vi "libssh2_session_callback_set.vi"(8 "error in (no error)":errorcluster, 9 "callback (0 = use built-in)":u64, 10 "callback type":T1, 11 "session":T2) -> (0 "error out":errorcluster, 2 "previous callback":u64)   [LabVIEW 2017, in "libssh2.lvlib"]
doc: "<B>DEPRECATED</B> (libssh2-1.11.1, use libssh2_session_callback_set2.vi)\n\nSet a callback handler for a session. Callbacks are triggered by the receipt of special packets at the transport layer.\n\nSet <B>callback</B> to 0 to to use the built-in default callback handler of lvssh2 (only available when the extension library is enabled). When the extension library is disabled, setting <B>callback</B> to 0 will disable the callback handler."
uses:
  libssh2.lvlib
  Session Refnum.ctl
  libssh2_session_callback_type.ctl
  Not A Session.vi
  <vilib>/Utility/error.llb/Error Cluster From Error Code.vi
  Global Settings.vi
  Read Session Refnum.vi
  <vilib>/Utility/semaphor.llb/Acquire Semaphore.vi
  <vilib>/Utility/semaphor.llb/Release Semaphore.vi
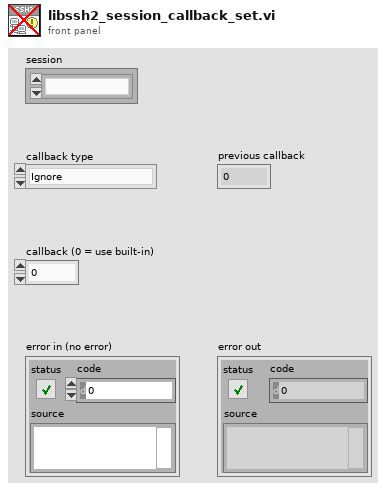
[diagram p1: front panel]
types:
  T1 = typedef "libssh2.lvlib/libssh2_session_callback_type.ctl" = enum16{"Ignore", "Debug", "Disconnect", "MAC Error", "X11", "Send", "Receive", "Auth Agent", "Auth Agent Identities", "Auth Agent Sign"}
  T2 = typedef "libssh2.lvlib/Session Refnum.ctl" = refnum<k1>
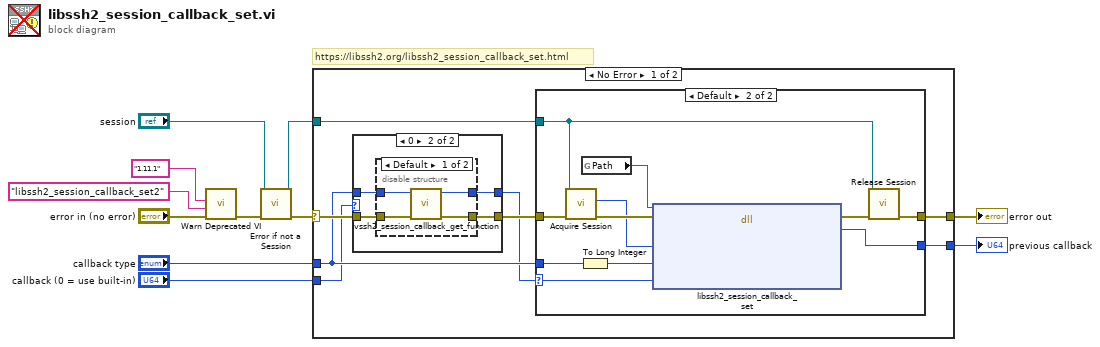
[diagram p0: block diagram]
diagram:
  # "https://libssh2.org/libssh2_session_callback_set.html"
  n1 = call "Warn Deprecated VI.vi"("error in (no error)"="error in (no error)", "replacement"="libssh2_session_callback_set2", "deprecated version"="1.11.1") -> ("error out"=w1:errorcluster)  [unwired: 8 in]
  n2 = call "Error if not a Session.vi"("error in (no error)"=w1, "session"="session") -> ("error out"=w6:errorcluster, "session out"=w5:T2)  [unwired: 8 in]
  n3 = case shown="No Error" w6 {
    selector: w6 -> [w19 w44]
    tunnel: [w13 w44] -> w11
    tunnel: w5 -> [w12 _]
    tunnel: "callback type" -> [w17 _]
    tunnel: [w16 _] -> w8
    tunnel: "callback (0 = use built-in)" -> [w14 _]
    frame No Error {
      n4 = case shown="0" w14 {
        selector: w14 -> [w33 _]
        tunnel: w19 -> [w32 w37]
        tunnel: [w32 w36] -> w18
        tunnel: w17 -> [_ w35]
        tunnel: [w33 w34] -> w15
        frame Default {
        }
        frame 0 {
          n5 = disable-structure shown="Default" {
            disable-tunnel: w37 -> [w41 w42]
            disable-tunnel: [w40 w42] -> w36
            disable-tunnel: w35 -> [w39 w43]
            disable-tunnel: [w38 w43] -> w34
            frame condition #0 (active) {
              n6 = call "lvssh2_session_callback_get_function.vi"("error in (no error)"=w41, "callback type"=w39) -> ("error out"=w40:errorcluster, "callback function"=w38:u64)  [unwired: 8 in]
            }
            frame condition #1 {
            }
          }
        }
      }
      n7 = case shown="Default" w15 {
        selector: w15 -> [_ w23]
        tunnel: w18 -> [w20 w27]
        tunnel: w17 -> [_ w26]
        tunnel: [_ w24] -> w16
        tunnel: [w20 w22] -> w13
        tunnel: w12 -> [_ w21]
        frame 0 {
        }
        frame Default {
          n8 = call "Acquire Session.vi"("error in (no error)"=w27, "session"=w21) -> ("error out"=w31:errorcluster, "LIBSSH2_SESSION*"=w30:u64)  [unwired: 7 in, 1 out]
          n9 = To Long Integer(number=w26) -> (32bit integer=w28:i32)
          n10 = global read "Global Settings.vi" "Path"() -> (w29:path)
          n11 = dll-call lib="?" fn="libssh2_session_callback_set"(path in=w29, error in=w31, "session"=w30, "cbtype"=w28, "callback"=w23) -> (error out=w25:errorcluster, "return value"=w24:u64)  [unwired: 4 in, 1 out]
          n12 = call "Release Session.vi"("error in (no error)"=w25, "session"=w21) -> ("error out"=w22:errorcluster)  [unwired: 9 in]
        }
      }
    }
    frame Error {
    }
  }
  "error out" <- w11
  "previous callback" <- w8
